vi "RandomWalk.vi"(1 "Current Robot Position":i32[](array[numeric])) -> (0 "New Robot Position":i32[](array[numeric]))   [LabVIEW 2012]
panel:
  in  "Noise Level":i32=10
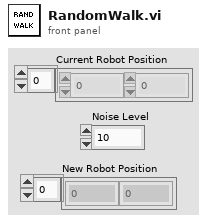
[diagram p1: front panel]
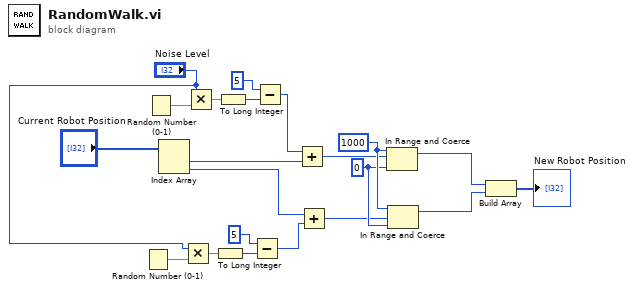
[diagram p0: block diagram]
diagram:
  w20 = 0 ("lower limit")
  w21 = 1000
  n1 = Random Number (0-1)() -> (number: 0 to 1=w7:dbl)
  n2 = Random Number (0-1)() -> (number: 0 to 1=w17:dbl)
  n3 = Index Array(array="Current Robot Position") -> (element #1=w15:i32, element #2=w2:i32)  [unwired: 2 in]
  n4 = Multiply(x="Noise Level", y=w7) -> (x*y=w6:dbl)
  n5 = Multiply(x="Noise Level", y=w17) -> (x*y=w16:dbl)
  n6 = To Long Integer(number=w6) -> (32bit integer=w5:i32)
  n7 = To Long Integer(number=w16) -> (32bit integer=w10:i32)
  n8 = Subtract(x=5, y=w5) -> (x-y=w1:i32)
  n9 = Subtract(x=5, y=w10) -> (x-y=w8:i32)
  n10 = Add(x=w8, y=w15) -> (x+y=w19:i32)
  n11 = Add(x=w2, y=w1) -> (x+y=w18:i32)
  n12 = In Range and Coerce(upper limit=w21, x=w19, lower limit=w20) -> (coerced(x)=w12:i32)  [unwired: 1 out]
  n13 = In Range and Coerce(upper limit=w21, x=w18, lower limit=w20) -> (coerced(x)=w11:i32)  [unwired: 1 out]
  n14 = Build Array(w12, w11) -> (→"New Robot Position":i32[])
